vi "FGV_CLIENT_error_buffer.vi"(4 "main_tab":refnum<vi>, 6 "thread":T1, 7 "option":T2=enum."display", 8 "error_in":errorcluster, 9 "error_indicator_global":refnum<vi>, 10 "error_indicator_tab":refnum<vi>, 11 "error_display_ref":refnum<vi>) -> (0 "error_out":errorcluster, 3 "error?":bool)   [LabVIEW 2019]
doc: "This VI check if error on error_in input is already in the buffer, and if not adds it to buffer and sends error event to event structure. VI also clears errors."
uses:
  FGV_CLIENT_error_buffer.ctl
  MAIN/thread_name.ctl
  <vilib>/Utility/miscctls.llb/LVRowAndColumnTypeDef.ctl
  <vilib>/Utility/miscctls.llb/LVRowAndColumnUnsignedTypeDef.ctl
  _misc/AULocalize/SubVIs/Get Localized Phrase Compact Interface 1D.vi
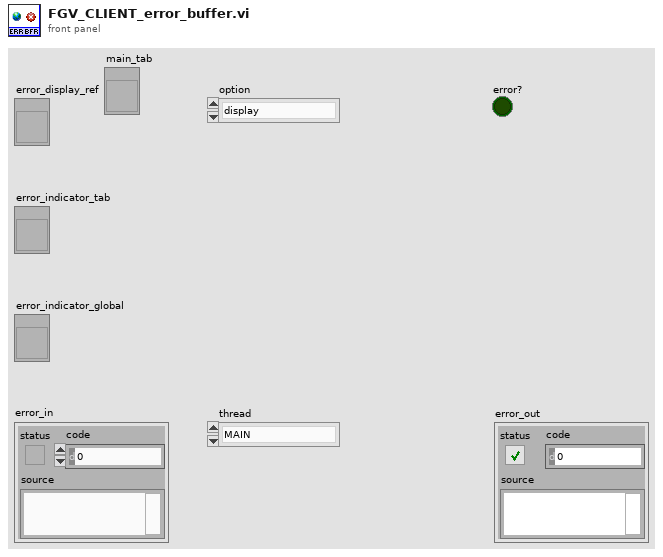
[diagram p1: front panel]
types:
  T1 = typedef "thread_name.ctl" = enum16{"MAIN"}
  T2 = typedef "FGV_CLIENT_error_buffer.ctl" = enum16{"initialize", "clear", "display", "get_status"}
  T3 = typedef "LVRowAndColumnUnsignedTypeDef.ctl" = cluster{"Row":u32, "Column":u32}
  T4 = typedef "LVRowAndColumnTypeDef.ctl" = cluster{"Row":i32, "Column":i32}
  T5 = enum32{"Reports", "Reference Editor", "Archivisation Editor", "User Management", "Manual SQL Requests", "Text SQL Requests", "Errors"}
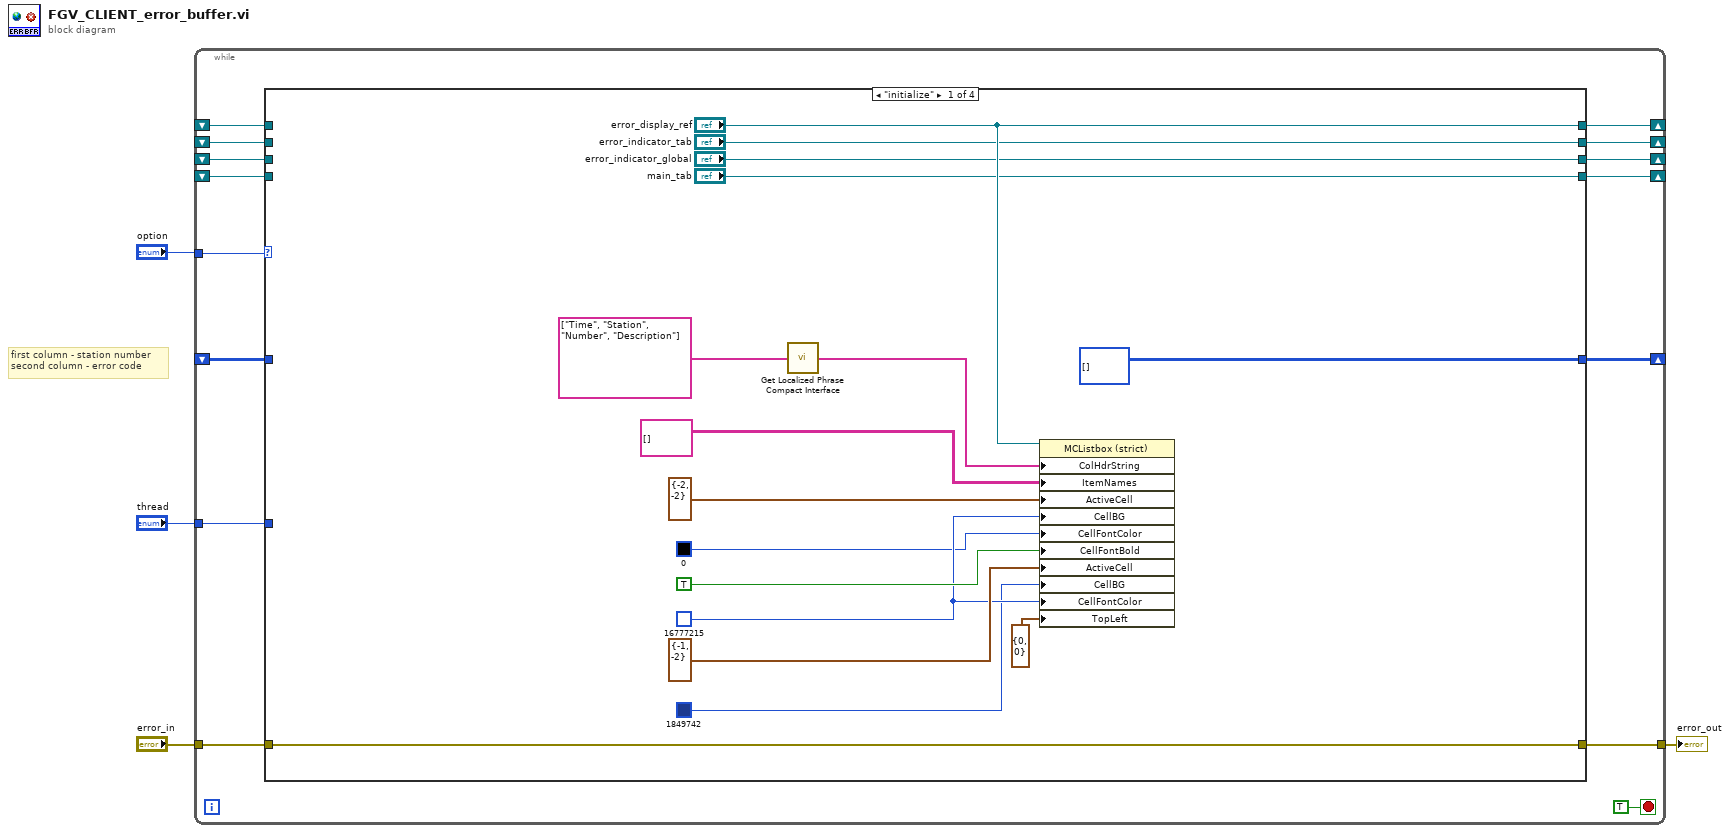
[diagram p0: block diagram]
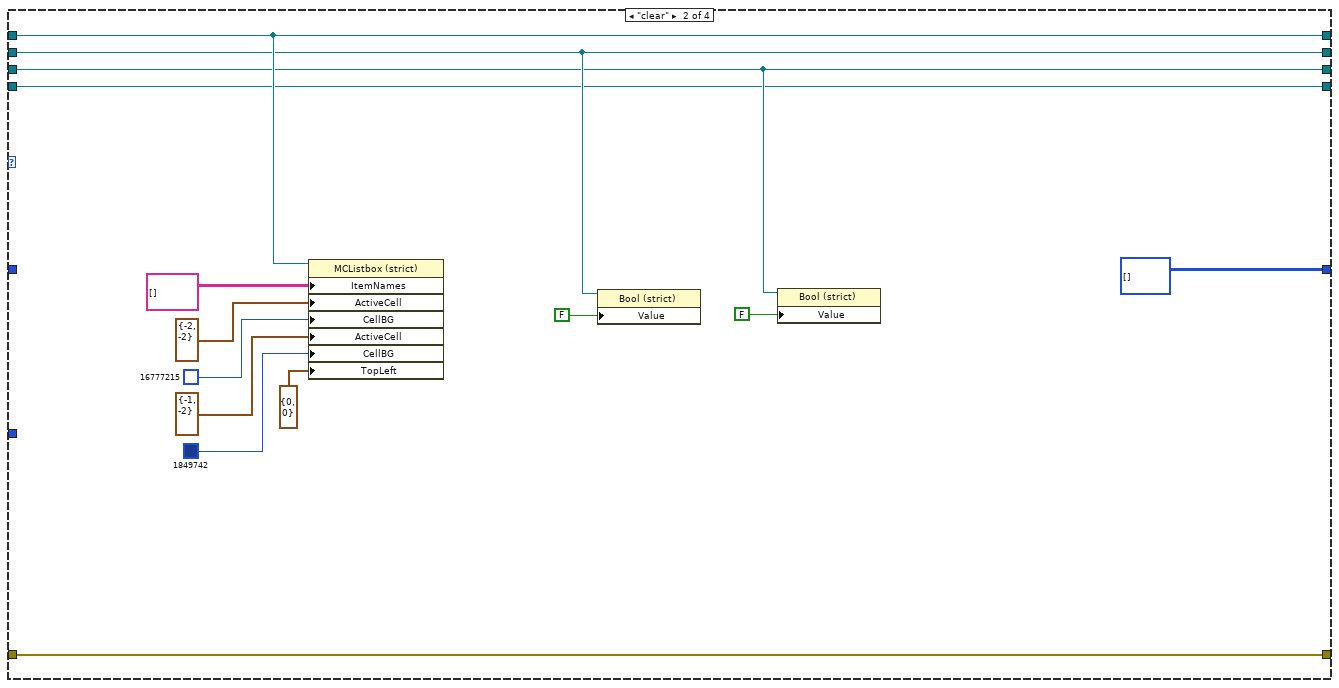
[diagram p2: hidden frame]
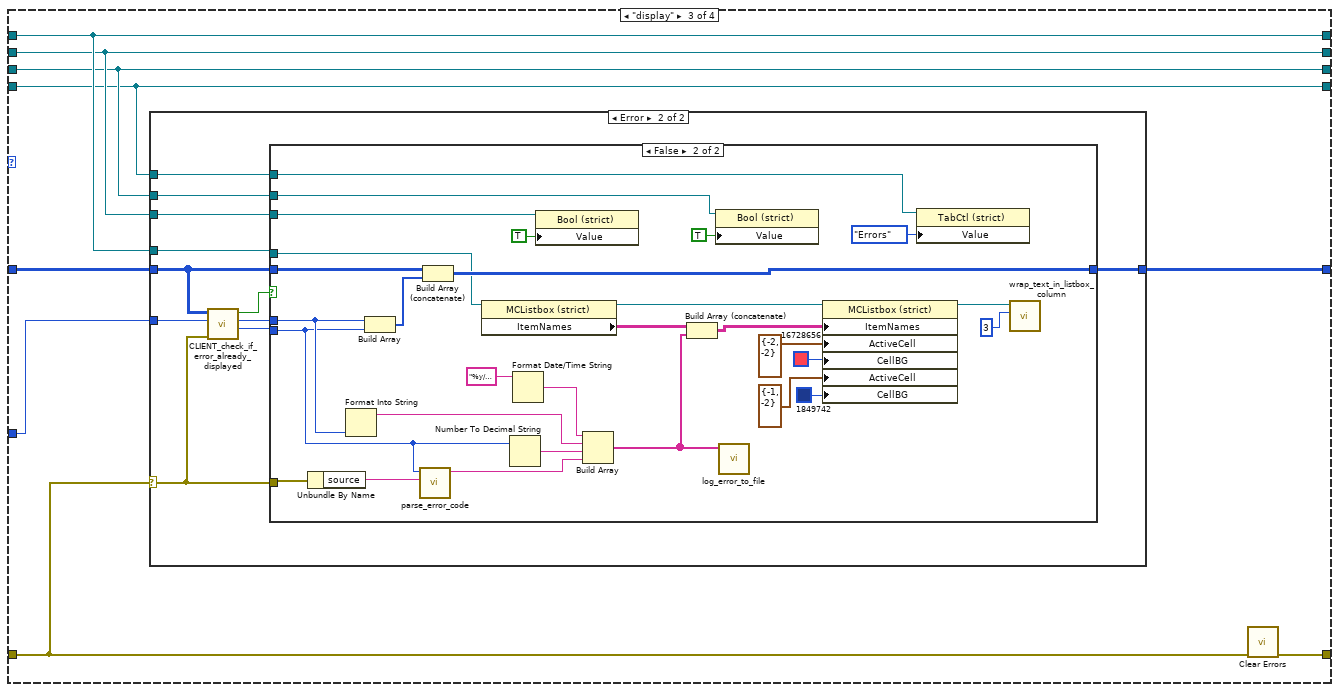
[diagram p3: hidden frame]
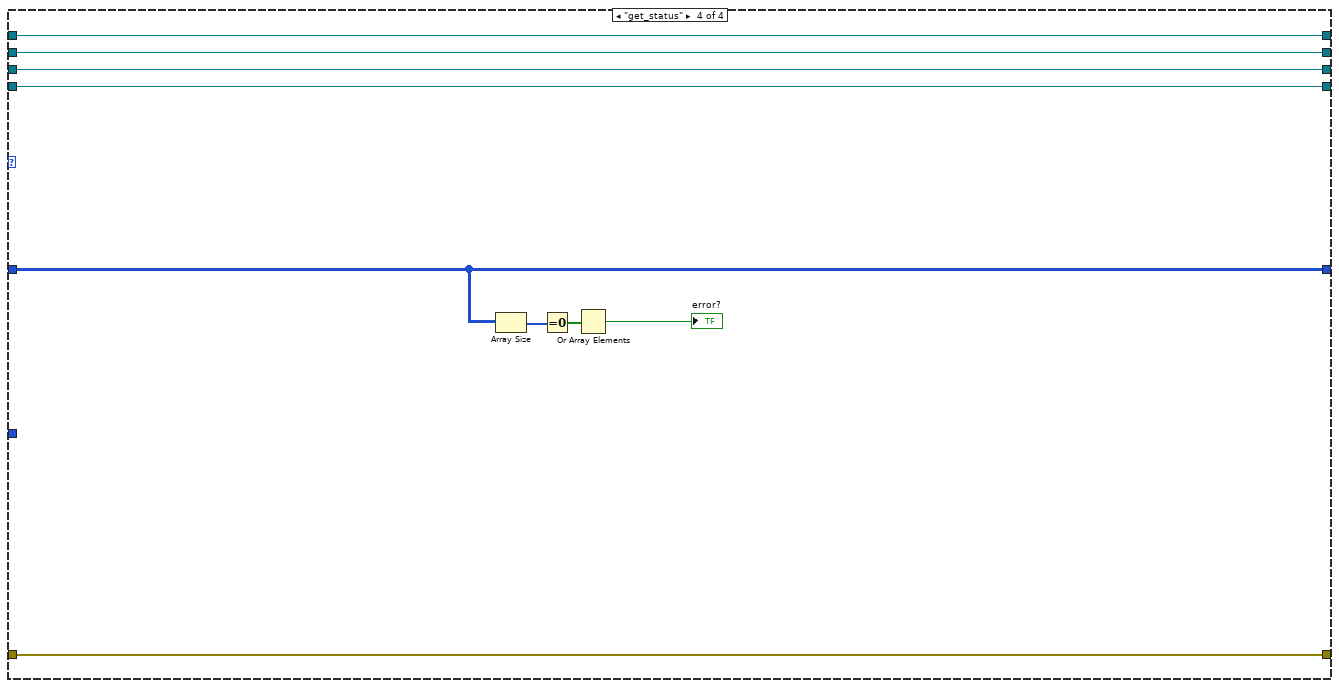
[diagram p6: hidden frame]
diagram:
  # "first column - station number\nsecond column - error code"
  n1 = while {
    tunnel: "option" -> [w18]
    tunnel: [w17] -> w4
    tunnel: "error_in" -> [w16]
    shift-right: [w15] -> _
    shift-left: _ -> [w14]
    shift-right: [w13] -> _
    shift-left: _ -> [w12]
    tunnel: "thread" -> [w11]
    shift-right: [w10] -> _
    shift-left: _ -> [w8]
    shift-right: [w9] -> _
    shift-left: _ -> [w7]
    shift-right: [w6] -> _
    shift-left: _ -> [w5]
    stop <- TRUE stop-if-true
    n2 = case shown="\"initialize\"" w18 {
      tunnel: [w35 w49 w57 w108] -> w17
      tunnel: w16 -> [w35 w49 w56 w108]
      tunnel: [i32[][] [] i32[][] [] w55 w109] -> w15
      tunnel: w14 -> [_ _ w58 w109]
      tunnel: ["error_display_ref" w42 w53 w107] -> w13
      tunnel: w12 -> [_ w42 w53 w107]
      tunnel: w11 -> [_ _ w54 _]
      tunnel: ["error_indicator_tab" w41 w52 w103] -> w10
      tunnel: ["error_indicator_global" w40 w51 w102] -> w9
      tunnel: w8 -> [_ w41 w52 w103]
      tunnel: w7 -> [_ w40 w51 w102]
      tunnel: ["main_tab" w37 w50 w101] -> w6
      tunnel: w5 -> [_ w37 w50 w101]
      frame "initialize" {
        w31 = u32 16777215
        n3 = call-poly "Get Localized Phrase Compact Interface.vi"("Key"=string[] ["Time", "Station", "Number", "Description"] ("Column Header Strings[]")) -> ("Translated Phrase"=w20:string[])
        n4 = property on="Property Node" class="MCListbox (strict)"(reference="error_display_ref", "ColHdrString"=w20, "ItemNames"=string[][] [] ("Item Names"), "ActiveCell"=T4 {"Row"=-2, "Column"=-2} ("Active Cell:Active Cell"), "CellBG"=w31, "CellFontColor"=u32 0, "CellFontBold"=TRUE ("Active Cell:Cell Font:Bold"), "ActiveCell"=T4 {"Row"=-1, "Column"=-2} ("Active Cell:Active Cell"), "CellBG"=u32 1849742, "CellFontColor"=w31, "TopLeft"=T3 {"Row"=0, "Column"=0} ("Top Left Visible Cell")) -> ()  [unwired: 1 in, 2 out]
      }
      frame "clear" {
        n5 = property on="Property Node" class="MCListbox (strict)"(reference=w42, "ItemNames"=string[][] [] ("Item Names"), "ActiveCell"=T4 {"Row"=-2, "Column"=-2} ("Active Cell:Active Cell"), "CellBG"=u32 16777215, "ActiveCell"=T4 {"Row"=-1, "Column"=-2} ("Active Cell:Active Cell"), "CellBG"=u32 1849742, "TopLeft"=T3 {"Row"=0, "Column"=0} ("Top Left Visible Cell")) -> ()  [unwired: 1 in, 2 out]
        n6 = property on="Property Node" class="Bool (strict)"(reference=w41, "Value"=FALSE) -> ()  [unwired: 1 in, 2 out]
        n7 = property on="Property Node" class="Bool (strict)"(reference=w40, "Value"=FALSE) -> ()  [unwired: 1 in, 2 out]
      }
      frame "display" {
        n8 = case shown="Error" w56 {
          selector: w56 -> [_ w63]
          tunnel: w58 -> [w59 w67]
          tunnel: [w59 w69] -> w55
          tunnel: w54 -> [_ w66]
          tunnel: w53 -> [_ w64]
          tunnel: w52 -> [_ w62]
          tunnel: w51 -> [_ w61]
          tunnel: w50 -> [_ w60]
          frame No Error {
          }
          frame Error {
            n9 = call "CLIENT_check_if_error_already_displayed.vi"("error_in"=w63, "thread_in"=w66, "displayed_errors"=w67) -> ("error_code"=w65:i32, "thread_out"=w68:T1, "already_displayed?"=w70:bool)  [unwired: 6 in]
            n10 = case shown="False" w70 {
              tunnel: w67 -> [w71 w99]
              tunnel: [w71 w100] -> w69
              tunnel: w68 -> [_ w93]
              tunnel: w65 -> [_ w82]
              tunnel: w64 -> [_ w97]
              tunnel: w63 -> [_ w91]
              tunnel: w62 -> [_ w77]
              tunnel: w61 -> [_ w76]
              tunnel: w60 -> [_ w73]
              frame True {
              }
              frame False {
                n11 = Unbundle By Name(w91) -> ("source"=w83:string)
                n12 = Format Into String(w93) -> (resulting string=w92:string)  [unwired: 3 in, 1 out]
                n13 = Build Array(w93, w82) -> (w98:i32[])
                n14 = call "parse_error_code.vi"("source"=w83, "code"=w82) -> ("parsed_error_string"=w81:string)  [unwired: 9 in]
                n15 = Build Array (concatenate)(w99, w98) -> (w100:i32[][])
                n16 = property class="MCListbox (strict)"(reference=w97) -> (reference out=w85:refnum<vi>, "ItemNames"=w90:string[][])  [unwired: 1 in, 1 out]
                n17 = Number To Decimal String(number=w82) -> (decimal integer string=w94:string)  [unwired: 1 in]
                n18 = Format Date/Time String(time format string (%c)="%y/%m/%d %H:%M:%S") -> (date/time string=w96:string)  [unwired: 2 in]
                n19 = property on="Property Node" class="Bool (strict)"(reference=w77, "Value"=TRUE) -> ()  [unwired: 1 in, 2 out]
                n20 = Build Array(w96, w92, w94, w81) -> (w80:string[])
                n21 = Build Array (concatenate)(w90, w80) -> (w84:string[][])
                n22 = property on="Property Node" class="Bool (strict)"(reference=w76, "Value"=TRUE) -> ()  [unwired: 1 in, 2 out]
                n23 = call "log_error_to_file.vi"("error_info"=w80) -> ()  [unwired: 11 in]
                n24 = property on="Property Node" class="MCListbox (strict)"(reference=w85, "ItemNames"=w84, "ActiveCell"=T4 {"Row"=-2, "Column"=-2} ("Active Cell:Active Cell"), "CellBG"=u32 16728656 ("Color Box"), "ActiveCell"=T4 {"Row"=-1, "Column"=-2} ("Active Cell:Active Cell"), "CellBG"=u32 1849742) -> (reference out=w75:refnum<vi>)  [unwired: 1 in, 1 out]
                n25 = property on="Property Node" class="TabCtl (strict)"(reference=w73, "Value"=T5."Errors") -> ()  [unwired: 1 in, 2 out]
                n26 = call "wrap_text_in_listbox_column.vi"("colum_to_wrap"=3, "multicolumn_listbox_reference"=w75) -> ()  [unwired: 8 in, 2 out]
              }
            }
          }
        }
        n27 = call <vilib>:"Clear Errors.vi"("error in (no error)"=w56) -> ("error out"=w57:errorcluster)  [unwired: 5 in, 1 out]
      }
      frame "get_status" {
        n28 = Array Size(array=w109) -> (size(s)=w106:i32[])
        n29 = Equal To 0?(x=w106) -> (x = 0?=w105:bool[])
        n30 = Or Array Elements(Boolean array=w105) -> (logical OR=→"error?":bool)
      }
    }
  }
  "error_out" <- w4
